vi "Traverse_Space.vi"(7 "Simulate/Run":T1=enum."Run VI", 9 "Show Panel?":bool, 10 "Traverse Setup":string) -> (3 "Error Comments":string)   [LabVIEW 2022 SP3]
doc: "This is an example of using features of the VI Server as a client. It shows how you might browse from one or more applications that may be exporting data from one or more data stations. \n\nThe example shows how to query a server for its list of exported VIs, how to get references to the VIs, and how call them with the Call By Reference function."
uses:
  Route mapping/Exclude_cluster.ctl
  Route mapping/Box_size.ctl
  Route mapping/Exclusion_type.ctl
  Controls/ok_button.ctl
  Controls/User_Specific_mode.ctl
  Globals/Constants_global.vi
  Globals/Trav_pos_global.vi
  Route mapping/Route_mapping_global.vi
panel:
  in  "Probe Support":T2=[{"Max"=15.0, "Min"=-15.0}, {"Max"=250.0, "Min"=0.0}, {"Max"=15.0, "Min"=-15.0}] {"Min" format="%#.1f"; "Max" format="%#.1f"}
  in  "Traverse space filename":u16(ring) items=["Default_Space_file.xls", "heelo.xls", "hello_test1.xls", "---Save As---"]
  in  "Traverse Name":u16(ring) items=["A_Tunnel", "A_Tunnel - Copy", "A_Tunnel_Turntable", "Aero_Enclosure", "Aero_Sting", "Aero_ThroughWall", "Aero_Tunnel", "Angle_Calibrator", "B_Tunnel", "D_Tunnel", "desktop", "dummy", "Dummy_Traverse", "EnFlo_Stack", "EnFlo_Trav1", "EnFlo_Trav3", "EnFlo_Trav4", "EnFlo_Tunnel", "EnFlo_Turntable", "F1_Wing_Angle", "Fast_Trav", "Fruit_Rig", "Hello_5.xls", "Laser_Disp_Scanner", "Laser_Meas_Traverse", "None", "Pitch_Traverse", "Pitch_Yaw", "PIV_Traverse", "Pressure_Port_1", "Pressure_Port_2", "Scanning Valve", "Soil_Rig", "Tank", "Trav_test"]
  out "Message":string
  in  "Cancel Button":bool
  in  "OK":T3
  in  "Traverse Limits":T2=[{"Max"=15001.0, "Min"=12000.0}, {"Max"=1000.0, "Min"=-1000.0}, {"Max"=700.0, "Min"=0.0}] {"Min" format="%#.1f"; "Max" format="%#.1f"}
  in  "Probe Volume":T2=[{"Max"=15.0, "Min"=-15.0}, {"Max"=250.0, "Min"=0.0}, {"Max"=15.0, "Min"=-15.0}] {"Min" format="%#.1f"; "Max" format="%#.1f"}
  in  "Exclude Array":T4[](array[typedef])=[{"Sizes"=[{"Max"=15000.0, "Min"=0.0}, {"Max"=1000.0, "Min"=-1000.0}, {"Max"=300.0, "Min"=0.0}], "Name"="Roughness Elements", "Exclude Type"=enum."Allow only vertical moves"}, {"Sizes"=[{"Max"=17000.0, "Min"=16000.0}, {"Max"=200.0, "Min"=-200.0}, {"Max"=-50.0, "Min"=-250.0}], "Name"="B204", "Exclude Type"=enum."Exclude completely"}] {"Sizes"."Min" format="%#.1f"; "Sizes"."Max" format="%#.1f"}
  # "Enter all coordinates assuming the Model Orientation is zero degrees"
  # "(Relative to measurement position)"
  # "X                           Y                          Z"
  # "X                           Y                          Z"
  # "(Relative to measurement position)"
  # "(Relative to measurement position)"
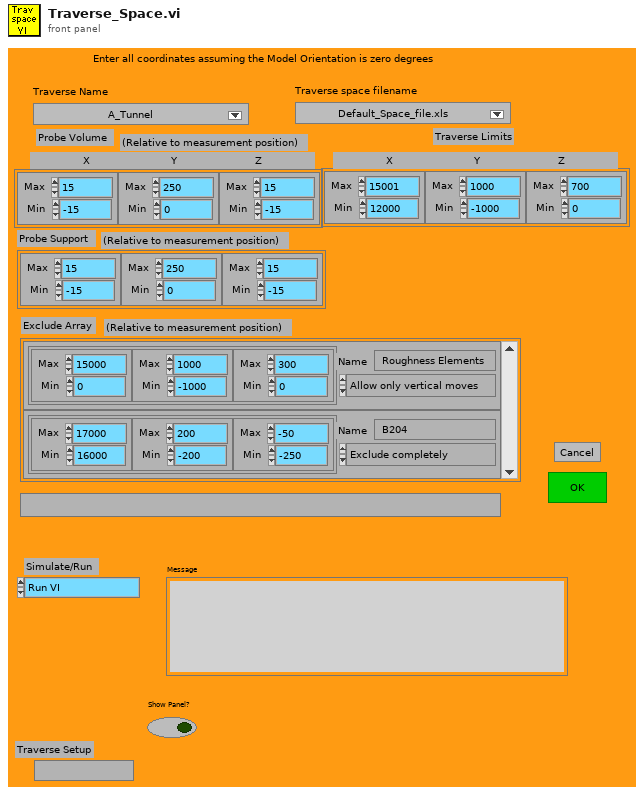
[diagram p1: front panel]
types:
  T1 = typedef "User_Specific_mode.ctl" = enum16{"Check VI only", "Run VI"}
  T2 = typedef "Box_size.ctl" = cluster{"Max":sgl, "Min":sgl}[]
  T3 = typedef "ok_button.ctl" = bool
  T4 = typedef "Exclude_cluster.ctl" = cluster{"Sizes":T2, "Name":string, "Exclude Type":T5}
  T5 = typedef "Exclusion_type.ctl" = enum16{"Exclude completely", "Allow only vertical moves"}
  T6 = enum16{"Load setup from excel file", "Save setup to excel file"}
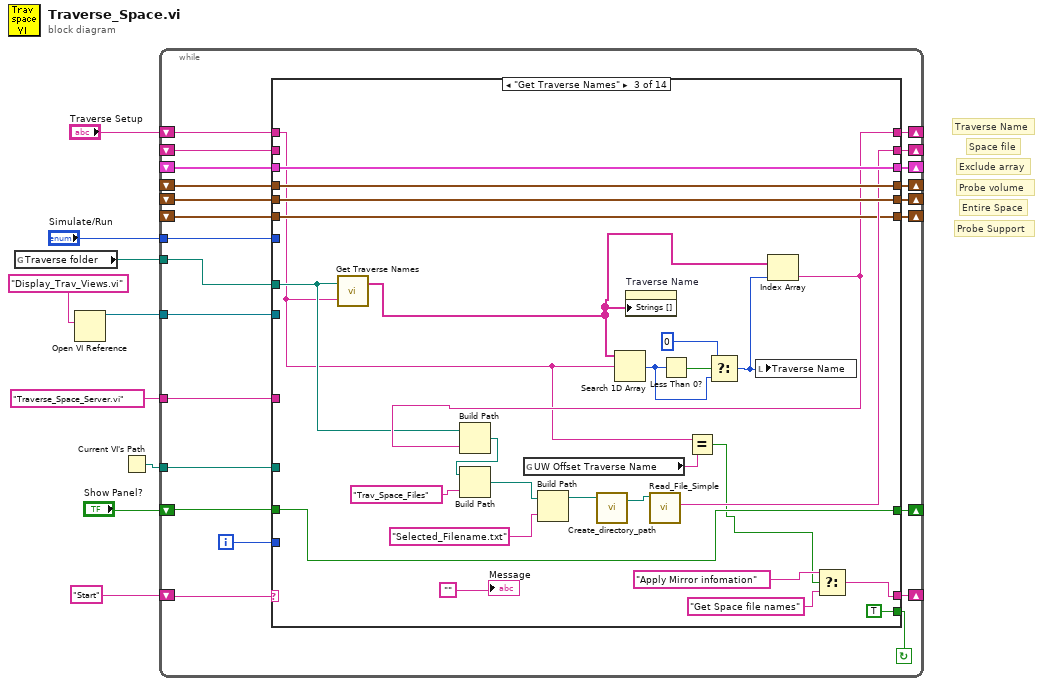
[diagram p0: block diagram]
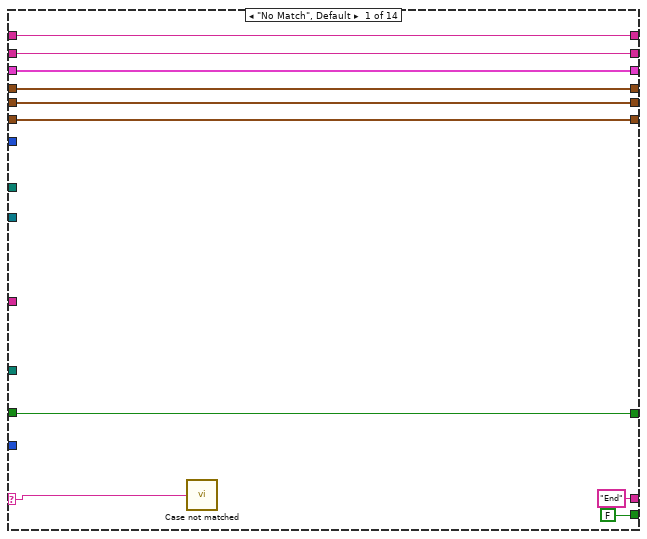
[diagram p2: hidden frame]
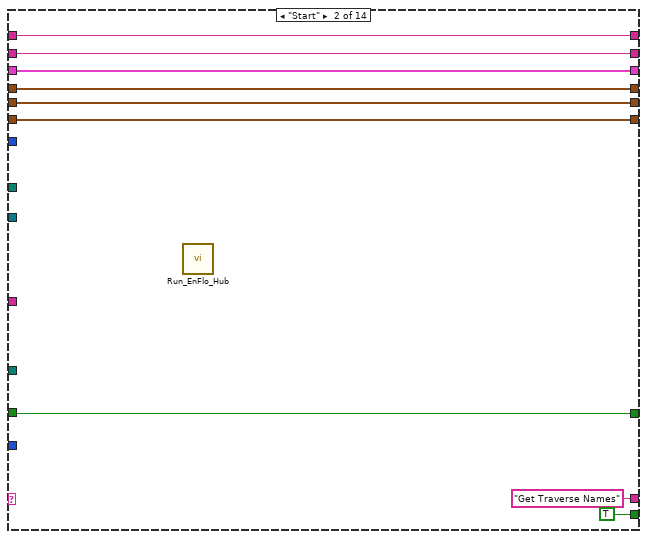
[diagram p3: hidden frame]
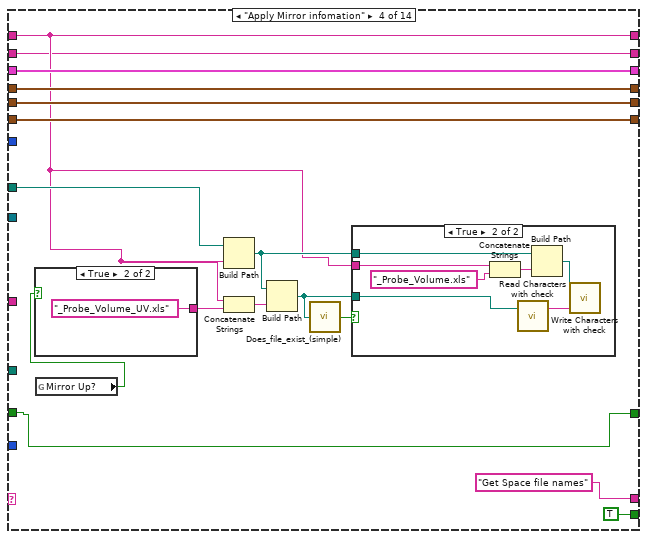
[diagram p4: hidden frame]
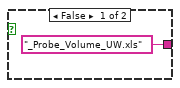
[diagram p6: hidden frame]
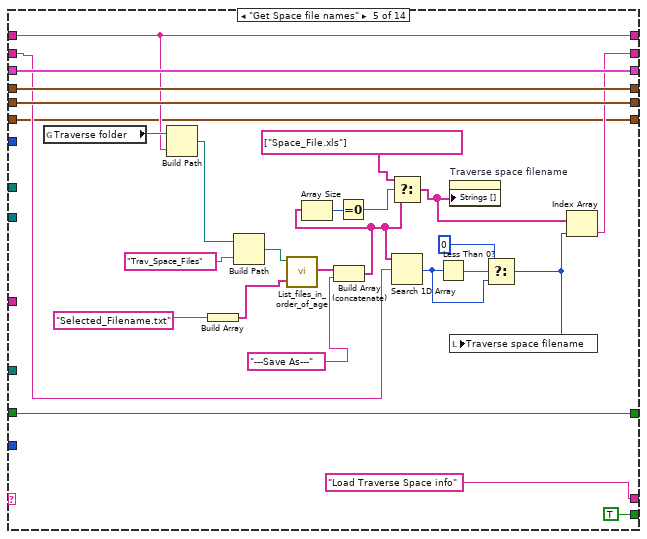
[diagram p7: hidden frame]
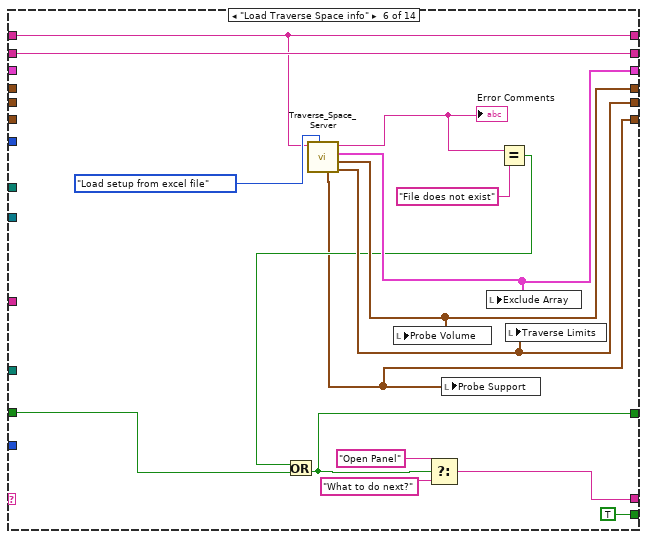
[diagram p8: hidden frame]
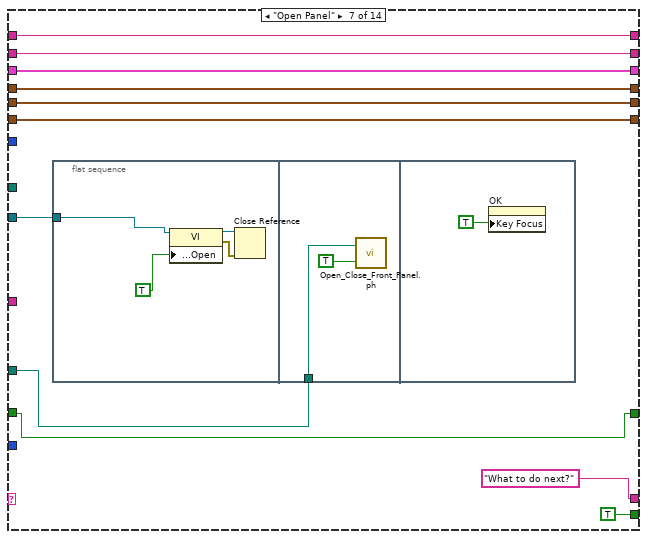
[diagram p9: hidden frame]
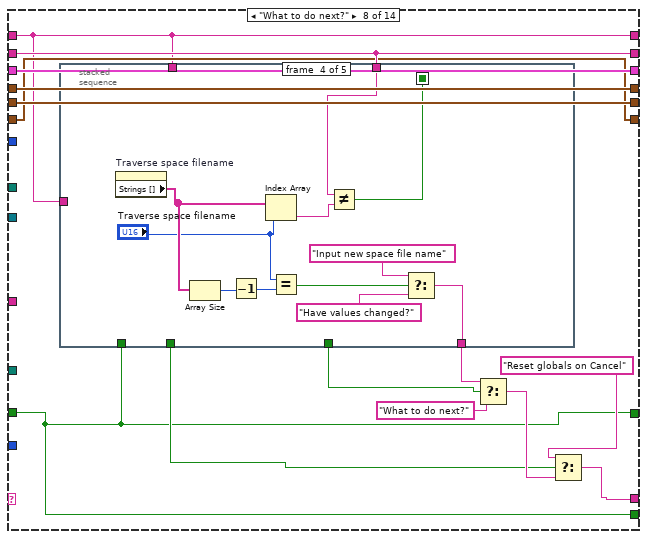
[diagram p10: hidden frame]
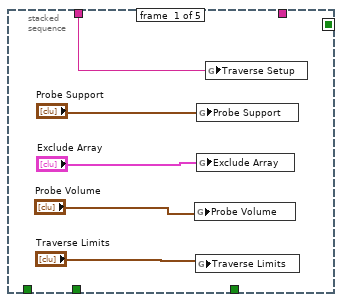
[diagram p11: hidden frame]
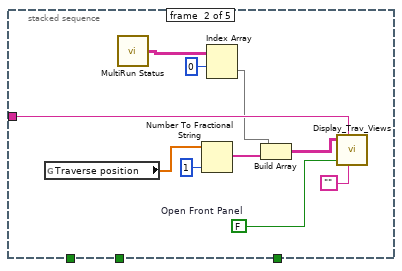
[diagram p12: hidden frame]
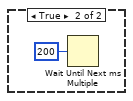
[diagram p14: hidden frame]
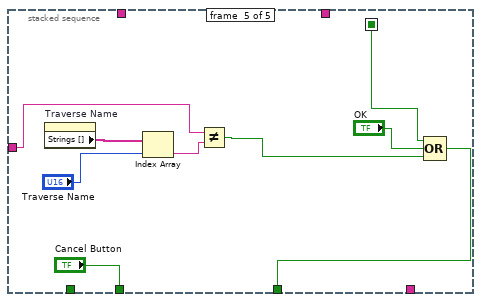
[diagram p15: hidden frame]
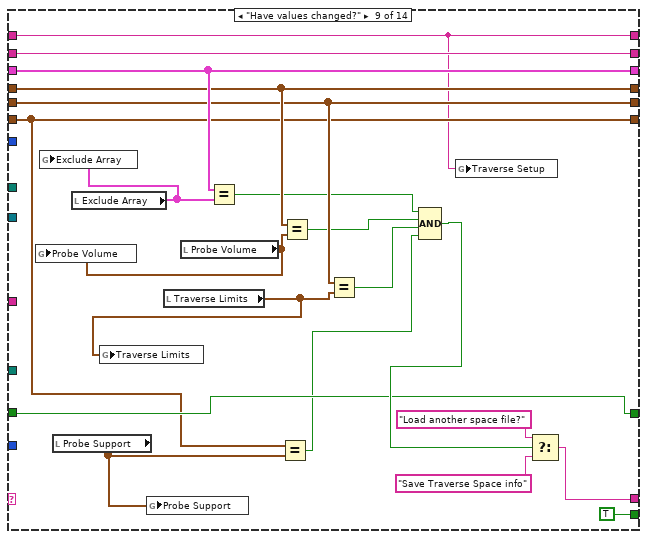
[diagram p16: hidden frame]
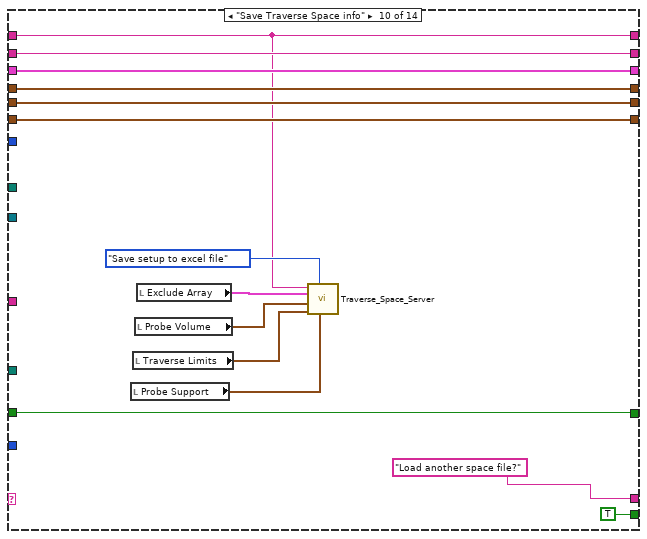
[diagram p17: hidden frame]
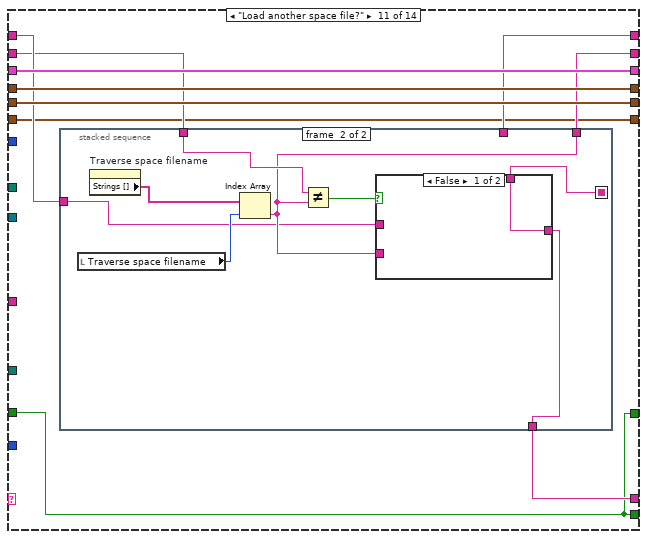
[diagram p18: hidden frame]
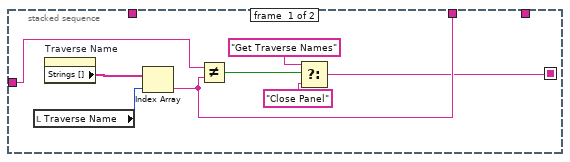
[diagram p19: hidden frame]
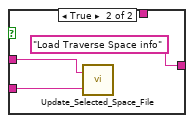
[diagram p20: hidden frame]
diagram:
  # "Probe Support"
  # "Traverse Name"
  # "Space file"
  # "Entire Space"
  # "Probe volume"
  # "Exclude array"
  n1 = global read "Constants_global.vi" "Traverse folder"() -> (w1:path)
  n2 = Open VI Reference(vi path="Display_Trav_Views.vi") -> (vi reference=w3:refnum<vi>)  [unwired: 1 in, 5 out]
  n3 = Current VI's Path() -> (path=w7:path)
  n4 = while {
    tunnel: "Traverse_Space_Server.vi" ("VI name to run on server") -> [w30]
    shift-left: "Start" -> [w27]
    shift-right: [w29] -> _
    tunnel: w7 -> [w28]
    shift-right: [w26] -> _
    shift-left: _ -> [w23]
    shift-right: [w25] -> _
    shift-left: _ -> [w22]
    shift-right: [w24] -> _
    shift-left: _ -> [w21]
    shift-right: [w19] -> _
    shift-left: "Traverse Setup" -> [w17]
    shift-right: [w20] -> _
    shift-left: _ -> [w18]
    shift-right: [w15] -> _
    shift-left: "Show Panel?" -> [w16]
    tunnel: w3 -> [w14]
    shift-right: [w13] -> _
    shift-left: _ -> [w12]
    tunnel: "Simulate/Run" -> [w11]
    tunnel: w1 -> [w10]
    i -> [w32]
    stop <- w31 continue-if-true
    n5 = case shown="\"Get Traverse Names\"" w27 {
      tunnel: w32 -> [_ _ _ _ _ _ _ _ _ _ _ _ _ _]
      tunnel: [FALSE ("status") TRUE ("status") TRUE ("status") TRUE ("status") TRUE ("status") TRUE ("status") TRUE ("status") w165 TRUE ("status") TRUE ("status") w251 w283 TRUE ("status") FALSE ("status")] -> w31
      selector: w27 -> [w33 _ _ _ _ _ _ _ _ _ _ _ _ _]
      tunnel: ["End" ("f") "Get Traverse Names" ("f") w58 "Get Space file names" "Load Traverse Space info" w145 "What to do next?" w177 w225 "Load another space file?" w252 w284 "Close Panel" "End"] -> w29
      tunnel: w30 -> [_ _ _ _ _ _ _ _ _ _ _ _ _ _]
      tunnel: w16 -> [w35 w44 w62 w88 w105 w135 w149 w165 w223 w239 w251 w283 w308 w320]
      tunnel: w28 -> [_ _ _ _ _ _ w152 _ _ _ _ _ _ w334]
      tunnel: [w40 w51 w77 w93 w128 w144 w155 w175 w235 w247 w259 w292 w313 w333] -> w26
      tunnel: [w39 w50 w76 w92 w127 w143 w154 w174 w234 w246 w258 w291 w312 w332] -> w25
      tunnel: [w38 w49 w75 w91 w126 w142 w153 w173 w233 w245 w257 w290 w311 w331] -> w24
      tunnel: w23 -> [w40 w51 w77 w93 w128 _ w155 w175 w235 w247 w259 w292 w313 w333]
      tunnel: w22 -> [w39 w50 w76 w92 w127 _ w154 w174 w234 w246 w258 w291 w312 w332]
      tunnel: w21 -> [w38 w49 w75 w91 w126 _ w153 w173 w233 w245 w257 w290 w311 w331]
      tunnel: [w36 w45 w63 w80 w111 w138 w150 w170 w224 w240 w253 w286 w309 w321] -> w20
      tunnel: [w37 w46 w60 w81 w110 w131 w151 w166 w216 w236 w255 w280 w306 w326] -> w19
      tunnel: w18 -> [w36 w45 _ w80 w109 w138 w150 w170 w224 w240 w254 w281 w309 w321]
      tunnel: w17 -> [w37 w46 w52 w81 w110 w131 w151 w166 w216 w236 w256 w280 w306 w326]
      tunnel: [w35 w44 w62 w88 w105 w133 w149 w165 w223 w239 w251 w283 w308 w320] -> w15
      tunnel: w14 -> [_ _ _ _ _ _ w148 _ _ _ _ _ _ w316]
      tunnel: [w34 w43 w61 w90 w104 w132 w147 w167 w218 w238 w250 w282 w307 w315] -> w13
      tunnel: w12 -> [w34 w43 w61 w90 w104 _ w147 w167 w218 w238 w250 w282 w307 w315]
      tunnel: w11 -> [_ _ _ _ _ _ _ _ _ _ _ _ _ _]
      tunnel: w10 -> [_ _ w54 w82 _ _ _ _ _ _ _ _ _ _]
      frame "No Match", Default {
        n6 = call "Case not matched.vi"("Case Name not Matched"=w33) -> ()
      }
      frame "Start" {
        n7 = call "Run_EnFlo_Hub.vi"() -> ()  [unwired: 1 in, 7 out]
      }
      frame "Get Traverse Names" {
        n8 = call "Get Traverse Names.vi"("Traverse name"=w52, "Traverse\nSetup\nFolder"=w54) -> ("Traverse Names"=w53:string[])  [unwired: 1 out]
        n9 = global read "Trav_pos_global.vi" "UW Offset Traverse Name"() -> (w56:string)
        n10 = Search 1D Array(1D array=w53, element=w52) -> (index of element=w72:i32)  [unwired: 1 out]
        n11 = property on="Traverse Name" class="Ring (strict)"("Strings []"=w53) -> ()  [unwired: 2 in, 2 out]
        n12 = Less Than 0?(x=w72) -> (x < 0?=w73:bool)
        n13 = Equal?(x=w52, y=w56) -> (x = y?=w55:bool)
        n14 = Select(t=0, s=w73, f=w72) -> (s? t:f=w70:i32)
        n15 = local write "Traverse Name"(w70) -> ()
        n16 = Index Array(array=w53, index=w70) -> (element=w60:string)
        n17 = Build Path(base path=w54, name or relative path=w60) -> (appended path=w68:path)
        n18 = Build Path(base path=w68, name or relative path="Trav_Space_Files" ("Substring")) -> (appended path=w67:path)
        n19 = Build Path(base path=w67, name or relative path="Selected_Filename.txt" ("Substring")) -> (appended path=w64:path)
        n20 = call "Create_directory_path.vi"("Path name"=w64) -> ("Path name Out"=w65:path)  [unwired: 2 in, 1 out]
        n21 = call "Read_File_Simple.vi"("Filename"=w65) -> ("string"=w63:string)  [unwired: 2 in, 7 out]
        n22 = Select(t="Apply Mirror infomation", s=w55, f="Get Space file names") -> (s? t:f=w58:string)
        "Message" <- ""
      }
      frame "Apply Mirror infomation" {
        n23 = global read "Trav_pos_global.vi" "Mirror Up?"() -> (w79:bool)
        n24 = case shown="True" w79 {
          tunnel: ["_Probe_Volume_UW.xls" ("string") "_Probe_Volume_UV.xls" ("string")] -> w84
          frame False {
          }
          frame True {
          }
        }
        n25 = Build Path(base path=w82, name or relative path=w81) -> (appended path=w86:path)
        n26 = Concatenate Strings(w81, w84) -> (w83:string)
        n27 = Build Path(base path=w86, name or relative path=w83) -> (appended path=w87:path)
        n28 = call "Does_file_exist_(simple).vi"("Pathname"=w87) -> ("exists?"=w85:bool)
        n29 = case shown="True" w85 {
          tunnel: w81 -> [_ w100]
          tunnel: w86 -> [_ w99]
          tunnel: w87 -> [_ w97]
          frame False {
          }
          frame True {
            n30 = Concatenate Strings(w100, "_Probe_Volume.xls" ("string")) -> (w98:string)
            n31 = call "Read Characters with check.vi"("file (use dialog)"=w97) -> ("Read String"=w95:string)  [unwired: 1 in, 1 out]
            n32 = Build Path(base path=w99, name or relative path=w98) -> (appended path=w96:path)
            n33 = call "Write Characters with check.vi"("String to Write"=w95, "file (use dialog)"=w96) -> ()  [unwired: 2 in, 1 out]
          }
        }
      }
      frame "Get Space file names" {
        n34 = global read "Constants_global.vi" "Traverse folder"() -> (w122:path)
        n35 = Build Path(base path=w122, name or relative path=w110) -> (appended path=w120:path)
        n36 = Build Array("Selected_Filename.txt" ("Substring")) -> (w119:string[])
        n37 = Build Path(base path=w120, name or relative path="Trav_Space_Files" ("Substring")) -> (appended path=w112:path)
        n38 = call "List_files_in_order_of_age.vi"("Files to Hide"=w119, "Folder"=w112) -> ("file names"=w108:string[])  [unwired: 9 in]
        n39 = Build Array (concatenate)(w108, "---Save As---") -> (w107:string[])
        n40 = Array Size(array=w107) -> (size(s)=w117:i32)
        n41 = Equal To 0?(x=w117) -> (x = 0?=w116:bool)
        n42 = Select(t=string[] ["Space_File.xls"] ("appended array"), s=w116, f=w107) -> (s? t:f=w114:string[])
        n43 = Search 1D Array(1D array=w107, element=w109) -> (index of element=w124:i32)  [unwired: 1 out]
        n44 = Less Than 0?(x=w124) -> (x < 0?=w125:bool)
        n45 = property on="Traverse space filename" class="Ring (strict)"("Strings []"=w114) -> ()  [unwired: 2 in, 2 out]
        n46 = Select(t=0, s=w125, f=w124) -> (s? t:f=w113:i32)
        n47 = local write "Traverse space filename"(w113) -> ()
        n48 = Index Array(array=w114, index=w113) -> (element=w111:string)
      }
      frame "Load Traverse Space info" {
        n49 = call "Traverse_Space_Server.vi"("Mode"=T6."Load setup from excel file", "Traverse Name"=w131) -> ("Traverse Limits Out"=w142:T2, "Probe Volume Out"=w143:T2, "Exclude Array Out"=w144:T4[], "Error Comments"=w136:string, "Probe Support Out"=w132:T2)  [unwired: 4 in, 1 out]
        "Error Comments" <- w136
        n50 = local write "Probe Volume"(w143) -> ()
        n51 = local write "Probe Support"(w132) -> ()
        n52 = local write "Exclude Array"(w144) -> ()
        n53 = Equal?(x=w136, y="File does not exist") -> (x = y?=w134:bool)
        n54 = Or(x=w134, y=w135) -> (x .or. y?=w133:bool)
        n55 = Select(t="Open Panel", s=w133, f="What to do next?") -> (s? t:f=w145:string)
        n56 = local write "Traverse Limits"(w142) -> ()
      }
      frame "Open Panel" {
        n57 = flat-sequence {
          tunnel: w148 -> [w158]
          tunnel: w152 -> [w162]
          frame #0 {
            n58 = property class="VI"(reference=w158, "Front Panel Window:Open"=TRUE) -> (reference out=w160:refnum<vi>, error out=w159:errorcluster)  [unwired: 1 in]
            n59 = Close Reference(reference=w160, error in (no error)=w159) -> ()  [unwired: 1 out]
          }
          frame #1 {
            n60 = call "Open_Close_Front_Panel.ph.vi"("openWindow (T)"=TRUE ("Front Panel Window:Open"), "VI path"=w162) -> ()  [unwired: 1 in, 1 out]
          }
          frame #2 {
            n61 = property on="OK" class="Bool"("Key Focus"=TRUE) -> ()  [unwired: 2 in, 2 out]
          }
        }
      }
      frame "What to do next?" {
        n62 = stacked-sequence {
          seq-local: [_ _ _ w200 _] -> [_ _ _ _ w207]
          tunnel: w166 -> [_ w191 _ _ w212]
          tunnel: [_ _ _ _ w208] -> w172
          tunnel: [_ _ _ _ "Cancel Button"] -> w171
          tunnel: w170 -> [_ _ _ w201 _]
          tunnel: [_ _ _ w197 _] -> w168
          tunnel: w166 -> [w179 _ _ _ _]
          tunnel: w165 -> [_ _ w194 _ _]
          frame #0 {
            n63 = global write "Route_mapping_global.vi" "Probe Volume"("Probe Volume") -> ()
            n64 = global write "Route_mapping_global.vi" "Traverse Limits"("Traverse Limits") -> ()
            n65 = global write "Route_mapping_global.vi" "Probe Support"("Probe Support") -> ()
            n66 = global write "Route_mapping_global.vi" "Exclude Array"("Exclude Array") -> ()
            n67 = global write "Route_mapping_global.vi" "Traverse Setup"(w179) -> ()
          }
          frame #1 {
            w192 = FALSE  # Open Front Panel
            n68 = global read "Trav_pos_global.vi" "Traverse position"() -> (w188:sgl[])
            n69 = call "MultiRun Status.vi"() -> ("Table Control"=w184:string[][])  [unwired: 1 in]
            n70 = Number To Fractional String(number=w188, precision (6)=i16 1) -> (F-format string=w187:string[])  [unwired: 2 in]
            n71 = Index Array(array=w184, index (row)=0) -> (element=w186:string[])  [unwired: 1 in]
            n72 = Build Array(w186, w187) -> (w185:string[][])
            n73 = call "Display_Trav_Views.vi"("Probe Positions"=w185, "Traverse Name"=w191, "Open Front Panel"=w192, "Error Comments"="") -> ()  [unwired: 3 in, 4 out]
          }
          frame #2 {
            n74 = case shown="False" w194 {
              frame False {
              }
              frame True {
                n75 = Wait Until Next ms Multiple(millisecond multiple=u32 200) -> ()  [unwired: 1 out]
              }
            }
          }
          frame #3 {
            n76 = property on="Traverse space filename" class="Ring (strict)"() -> ("Strings []"=w203:string[])  [unwired: 2 in, 2 out]
            n77 = Array Size(array=w203) -> (size(s)=w205:i32)
            n78 = Decrement(x=w205) -> (x-1=w204:i32)
            n79 = Index Array(array=w203, index="Traverse space filename") -> (element=w206:string)
            n80 = Equal?(x="Traverse space filename", y=w204) -> (x = y?=w199:bool)
            n81 = Not Equal?(x=w201, y=w206) -> (x != y?=w200:bool)
            n82 = Select(t="Input new space file name" ("f"), s=w199, f="Have values changed?") -> (s? t:f=w197:string)
          }
          frame #4 {
            n83 = property on="Traverse Name" class="Ring (strict)"() -> ("Strings []"=w213:string[])  [unwired: 2 in, 2 out]
            n84 = Index Array(array=w213, index="Traverse Name") -> (element=w211:string)
            n85 = Not Equal?(x=w212, y=w211) -> (x != y?=w210:bool)
            n86 = Compound Arithmetic op=OR(w207, "OK", w210) -> (w208:T3)
          }
        }
        n87 = Select(t=w168, s=w172, f="What to do next?") -> (s? t:f=w178:string)
        n88 = Select(t="Reset globals on Cancel", s=w171, f=w178) -> (s? t:f=w177:string)
      }
      frame "Have values changed?" {
        n89 = local read "Probe Support"() -> (w219:T2)
        n90 = local read "Exclude Array"() -> (w222:T4[])
        n91 = global write "Route_mapping_global.vi" "Exclude Array"(w222) -> ()
        n92 = global write "Route_mapping_global.vi" "Probe Support"(w219) -> ()
        n93 = local read "Traverse Limits"() -> (w220:T2)
        n94 = global write "Route_mapping_global.vi" "Traverse Limits"(w220) -> ()
        n95 = local read "Probe Volume"() -> (w221:T2)
        n96 = global write "Route_mapping_global.vi" "Probe Volume"(w221) -> ()
        n97 = Equal?(x=w235, y=w222) -> (x = y?=w232:bool)
        n98 = Equal?(x=w218, y=w219) -> (x = y?=w217:bool)
        n99 = Equal?(x=w234, y=w221) -> (x = y?=w231:bool)
        n100 = Equal?(x=w233, y=w220) -> (x = y?=w230:bool)
        n101 = Compound Arithmetic op=AND(w232, w231, w230, w217) -> (w228:bool)
        n102 = global write "Route_mapping_global.vi" "Traverse Setup"(w216) -> ()
        n103 = Select(t="Load another space file?", s=w228, f="Save Traverse Space info") -> (s? t:f=w225:string)
      }
      frame "Save Traverse Space info" {
        n104 = local read "Probe Support"() -> (w237:T2)
        n105 = local read "Traverse Limits"() -> (w241:T2)
        n106 = local read "Probe Volume"() -> (w242:T2)
        n107 = local read "Exclude Array"() -> (w243:T4[])
        n108 = call "Traverse_Space_Server.vi"("Probe Support"=w237, "Mode"=T6."Save setup to excel file", "Traverse Limits"=w241, "Probe Volume"=w242, "Exclude Array"=w243, "Traverse Name"=w236) -> ()  [unwired: 6 out]
      }
      frame "Load another space file?" {
        n109 = stacked-sequence {
          seq-local: [w261 _] -> [_ w270]
          tunnel: w256 -> [w266 w268]
          tunnel: [w262 _] -> w255
          tunnel: [_ w273] -> w252
          tunnel: w254 -> [_ w272]
          tunnel: [_ w269] -> w253
          frame #0 {
            n110 = local read "Traverse Name"() -> (w260:u16)
            n111 = property on="Traverse Name" class="Ring (strict)"() -> ("Strings []"=w267:string[])  [unwired: 2 in, 2 out]
            n112 = Index Array(array=w267, index=w260) -> (element=w262:string)
            n113 = Not Equal?(x=w266, y=w262) -> (x != y?=w265:bool)
            n114 = Select(t="Get Traverse Names" ("f"), s=w265, f="Close Panel") -> (s? t:f=w261:string)
          }
          frame #1 {
            n115 = local read "Traverse space filename"() -> (w274:u16)
            n116 = property on="Traverse space filename" class="Ring (strict)"() -> ("Strings []"=w275:string[])  [unwired: 2 in, 2 out]
            n117 = Index Array(array=w275, index=w274) -> (element=w269:string)
            n118 = Not Equal?(x=w272, y=w269) -> (x != y?=w271:bool)
            n119 = case shown="False" w271 {
              tunnel: [w276 "Load Traverse Space info" ("f")] -> w273
              tunnel: w270 -> [w276 _]
              tunnel: w269 -> [_ w278]
              tunnel: w268 -> [_ w277]
              frame False {
              }
              frame True {
                n120 = call "Update_Selected_Space_File.vi"("Selected Space File Name"=w278, "Traverse Setup"=w277) -> ()  [unwired: 1 in]
              }
            }
          }
        }
      }
      frame "Input new space file name" {
        n121 = property on="Traverse space filename" class="Ring (strict)"() -> ("Strings []"=w285:string[])  [unwired: 2 in, 2 out]
        n122 = call "Input_String_Dialog.vi"("Message to user"="Please Enter a new  space file name") -> ("Ok Out"=w287:bool, "Output string"=w288:string)  [unwired: 1 in]
        n123 = case shown="True" w287 {
          tunnel: w288 -> [_ w301]
          tunnel: [w294 w296] -> w286
          tunnel: w281 -> [w294 _]
          tunnel: w285 -> [_ w297]
          tunnel: ["What to do next?" ("f") "Save Traverse Space info" ("f")] -> w284
          tunnel: w280 -> [_ w295]
          frame False {
          }
          frame True {
            n124 = call "Fast_string_Replace.vi"("Replace match with:"="_", "Input String"=w301, "matchThis"=" " ("regular expression")) -> ("Output String"=w302:string)  [unwired: 1 in, 1 out]
            n125 = local write "Traverse space filename"(0) -> ()
            n126 = call "Add_filename_suffix.vi"("Filename"=w302, "Suffix to add"=".xls") -> ("Filename out"=w296:string)  [unwired: 3 out]
            n127 = Build Array (concatenate)(w296, w297) -> (w300:string[])
            n128 = property on="Traverse space filename" class="Ring (strict)"("Strings []"=w300) -> ()  [unwired: 2 in, 2 out]
            n129 = call "Update_Selected_Space_File.vi"("Selected Space File Name"=w296, "Traverse Setup"=w295) -> ()  [unwired: 1 in]
          }
        }
      }
      frame "Reset globals on Cancel" {
        n130 = global write "Route_mapping_global.vi" "Traverse Limits"(w311) -> ()
        n131 = global write "Route_mapping_global.vi" "Probe Volume"(w312) -> ()
        n132 = global write "Route_mapping_global.vi" "Exclude Array"(w313) -> ()
        n133 = global write "Route_mapping_global.vi" "Traverse Setup"(w306) -> ()
        n134 = global write "Route_mapping_global.vi" "Probe Support"(w307) -> ()
      }
      frame "Close Panel" {
        w324 = FALSE  # append to file? (new file:F)
        w325 = FALSE  # advisory dialog? (display:T)
        n135 = global read "Constants_global.vi" "Traverse folder"() -> (w330:path)
        n136 = call "Open_Close_Front_Panel.ph.vi"("openWindow (T)"=FALSE ("Front Panel Window:Open"), "VI path"=w334) -> ()  [unwired: 1 in, 1 out]
        n137 = Build Path(base path=w330, name or relative path=w326) -> (appended path=w328:path)
        n138 = Build Path(base path=w328, name or relative path="Trav_Space_Files" ("Substring")) -> (appended path=w327:path)
        n139 = Build Path(base path=w327, name or relative path="Selected_Filename.txt" ("Substring")) -> (appended path=w322:path)
        n140 = property class="VI"(reference=w316, "Front Panel Window:Open"=FALSE) -> (reference out=w318:refnum<vi>, error out=w317:errorcluster)  [unwired: 1 in]
        n141 = Close Reference(reference=w318, error in (no error)=w317) -> ()  [unwired: 1 out]
        n142 = call "Write_Characters_To_File.vi"("file path (dialog if empty)"=w322, "advisory dialog? (display:T)"=w325, "character string"=w321, "append to file? (new file:F)"=w324) -> ()  [unwired: 1 in, 4 out]
      }
    }
  }
